vi "Agilent E364X Series Output DC Voltage with Tracking.vi"(0 "VISA resource name":refnum<visa-resource-name>, 1 "Current Limit (0 Amps)":dbl format="%.2p", 2 "OVP Limit (22.0 Volts)":dbl=22.0 format="%.2p", 3 "OVP Enabled (True)":bool=TRUE, 5 "Voltage Level (0.0 Volts)":dbl format="%.2p", 7 "Output Enabled (False)":bool, 11 "error in (no error)":errorcluster, 12 "Current Limit 2 (0 Amps)":dbl format="%.2p", 13 "OVP Limit 2 (22.0 Volts)":dbl=22.0 format="%.2p", 14 "OVP Enabled 2 (True)":bool=TRUE) -> ()   [LabVIEW 2013]
doc: "This VI configures the specifies power supply's channel to generate a DC voltage by taking the following steps:\n\n1) Configure current limit.\n\n2) Configure the over voltage protection.\n\n3) Configure the voltage level.\n\n4) Enable or disable the power output.\n\n5) Query the over voltage output state.\n\nNotes:\n\n(1) This VI takes a couple seconds to finish so that it may correctly get the current OVP value."
uses:
  <instrlib>/Agilent E364X Series/Agilent E364X Series.lvlib
panel:
  # "© 2005 National Instruments.  ALL RIGHTS RESERVED."
  # "Output 1"
  # "Output 2"
  # "For instructions,\nselect Show Context Help\nfrom the Help menu."
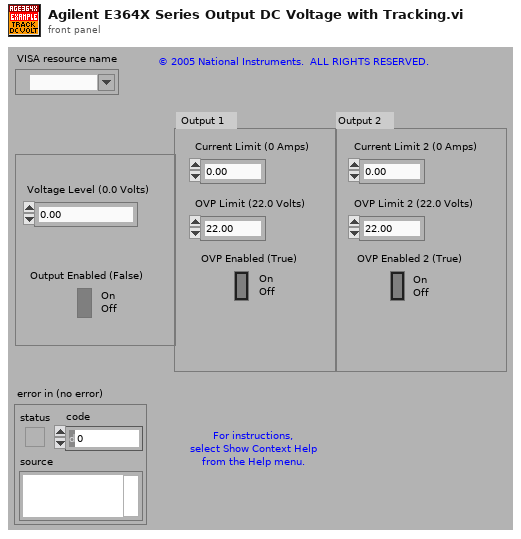
[diagram p1: front panel]
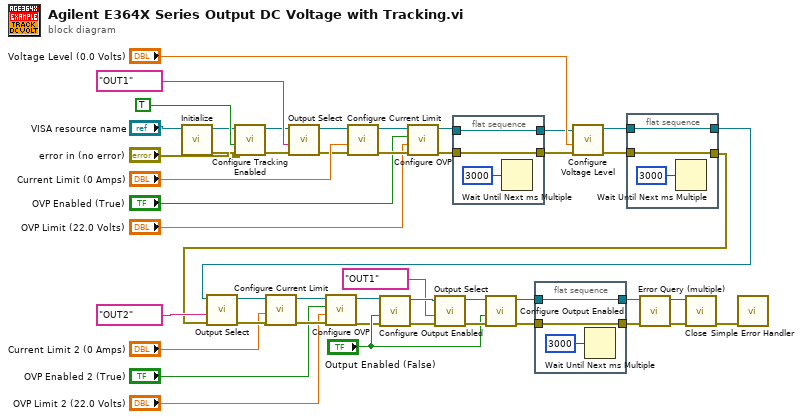
[diagram p0: block diagram]
diagram:
  n1 = call "Initialize.vi"("error in (no error)"="error in (no error)", "VISA resource name"="VISA resource name") -> ("error out"=w17:errorcluster, "VISA resource name out"=w16:refnum<visa-resource-name>)  [unwired: 8 in]
  n2 = call "Output Select.vi"("error in (no error)"=w9, "Instrument Select (Output 1)"="OUT2", "VISA resource name"=w11) -> ("error out"=w36:errorcluster, "VISA resource name out"=w37:refnum<visa-resource-name>)  [unwired: 7 in]
  n3 = call "Configure Tracking Enabled.vi"("error in (no error)"=w17, "Tracking Enabled (F: Off)"=TRUE ("Enabled (F: Off)"), "VISA resource name"=w16) -> ("error out"=w21:errorcluster, "VISA resource name out"=w22:refnum<visa-resource-name>)  [unwired: 7 in]
  n4 = call "Configure Current Limit.vi"("error in (no error)"=w36, "Current Limit (0.0 Amps)"="Current Limit 2 (0 Amps)", "VISA resource name"=w37) -> ("error out"=w34:errorcluster, "VISA resource name out"=w35:refnum<visa-resource-name>)  [unwired: 7 in]
  n5 = call "Output Select.vi"("error in (no error)"=w21, "Instrument Select (Output 1)"="OUT1", "VISA resource name"=w22) -> ("error out"=w40:errorcluster, "VISA resource name out"=w41:refnum<visa-resource-name>)  [unwired: 7 in]
  n6 = call "Configure OVP.vi"("error in (no error)"=w34, "Limit (22.0 Volts)"="OVP Limit 2 (22.0 Volts)", "OVP Enabled (T: On)"="OVP Enabled 2 (True)", "VISA resource name"=w35) -> ("error out"=w23:errorcluster, "VISA resource name out"=w24:refnum<visa-resource-name>)  [unwired: 6 in]
  n7 = call "Configure Current Limit.vi"("error in (no error)"=w40, "Current Limit (0.0 Amps)"="Current Limit (0 Amps)", "VISA resource name"=w41) -> ("error out"=w47:errorcluster, "VISA resource name out"=w46:refnum<visa-resource-name>)  [unwired: 7 in]
  n8 = call "Configure Output Enabled.vi"("error in (no error)"=w23, "Output Enabled (F: Off)"="Output Enabled (False)", "VISA resource name"=w24) -> ("error out"=w28:errorcluster, "VISA resource name out"=w30:refnum<visa-resource-name>)  [unwired: 7 in]
  n9 = call "Configure OVP.vi"("error in (no error)"=w47, "Limit (22.0 Volts)"="OVP Limit (22.0 Volts)", "OVP Enabled (T: On)"="OVP Enabled (True)", "VISA resource name"=w46) -> ("error out"=w2:errorcluster, "VISA resource name out"=w1:refnum<visa-resource-name>)  [unwired: 6 in]
  n10 = call "Output Select.vi"("error in (no error)"=w28, "Instrument Select (Output 1)"="OUT1", "VISA resource name"=w30) -> ("error out"=w27:errorcluster, "VISA resource name out"=w29:refnum<visa-resource-name>)  [unwired: 7 in]
  n11 = flat-sequence {
    tunnel: w1 -> [w49]
    tunnel: [w49] -> w4
    tunnel: w2 -> [w48]
    tunnel: [w48] -> w3
    frame #0 {
      n12 = Wait Until Next ms Multiple(millisecond multiple=u32 3000) -> ()  [unwired: 1 out]
    }
  }
  n13 = call "Configure Output Enabled.vi"("error in (no error)"=w27, "Output Enabled (F: Off)"="Output Enabled (False)", "VISA resource name"=w29) -> ("error out"=w5:errorcluster, "VISA resource name out"=w8:refnum<visa-resource-name>)  [unwired: 7 in]
  n14 = flat-sequence {
    tunnel: w8 -> [w52]
    tunnel: [w52] -> w7
    tunnel: [w51] -> w6
    tunnel: w5 -> [w51]
    frame #0 {
      n15 = Wait Until Next ms Multiple(millisecond multiple=u32 3000) -> ()  [unwired: 1 out]
    }
  }
  n16 = call "Configure Voltage Level.vi"("error in (no error)"=w3, "Level (0.0 Volts)"="Voltage Level (0.0 Volts)", "VISA resource name"=w4) -> ("error out"=w10:errorcluster, "VISA resource name out"=w12:refnum<visa-resource-name>)  [unwired: 7 in]
  n17 = flat-sequence {
    tunnel: w12 -> [w55]
    tunnel: [w55] -> w11
    tunnel: w10 -> [w54]
    tunnel: [w54] -> w9
    frame #0 {
      n18 = Wait Until Next ms Multiple(millisecond multiple=u32 3000) -> ()  [unwired: 1 out]
    }
  }
  n19 = call "Error Query (multiple).vi"("error in (no error)"=w6, "VISA resource name"=w7) -> ("error out"=w13:errorcluster, "VISA resource name out"=w14:refnum<visa-resource-name>)  [unwired: 6 in, 2 out]
  n20 = call "Close.vi"("error in (no error)"=w13, "VISA resource name"=w14) -> ("error out"=w15:errorcluster)  [unwired: 9 in]
  n21 = call <vilib>:"Simple Error Handler.vi"("error in (no error)"=w15) -> ()  [unwired: 4 in, 5 out]
